vi "Calculate Mean Histogram Y Values.vi"(11 "Histograms":u32[][](array[numeric])) -> (3 "Mean Row Values":u8[](array[numeric]))   [LabVIEW 2015]
uses:
  <userlib>/_OpenG.lib/array/array.llb/Sort 1D Array (U32)__ogtk.vi
  <vilib>/Analysis/NI_AALBase.lvlib
panel:
  out "Waveform Graph":u32[][](graph)
  out "number of columns":i32
  out "number of rows":i32
  out "Sorted Pointers":i32[](array[numeric])
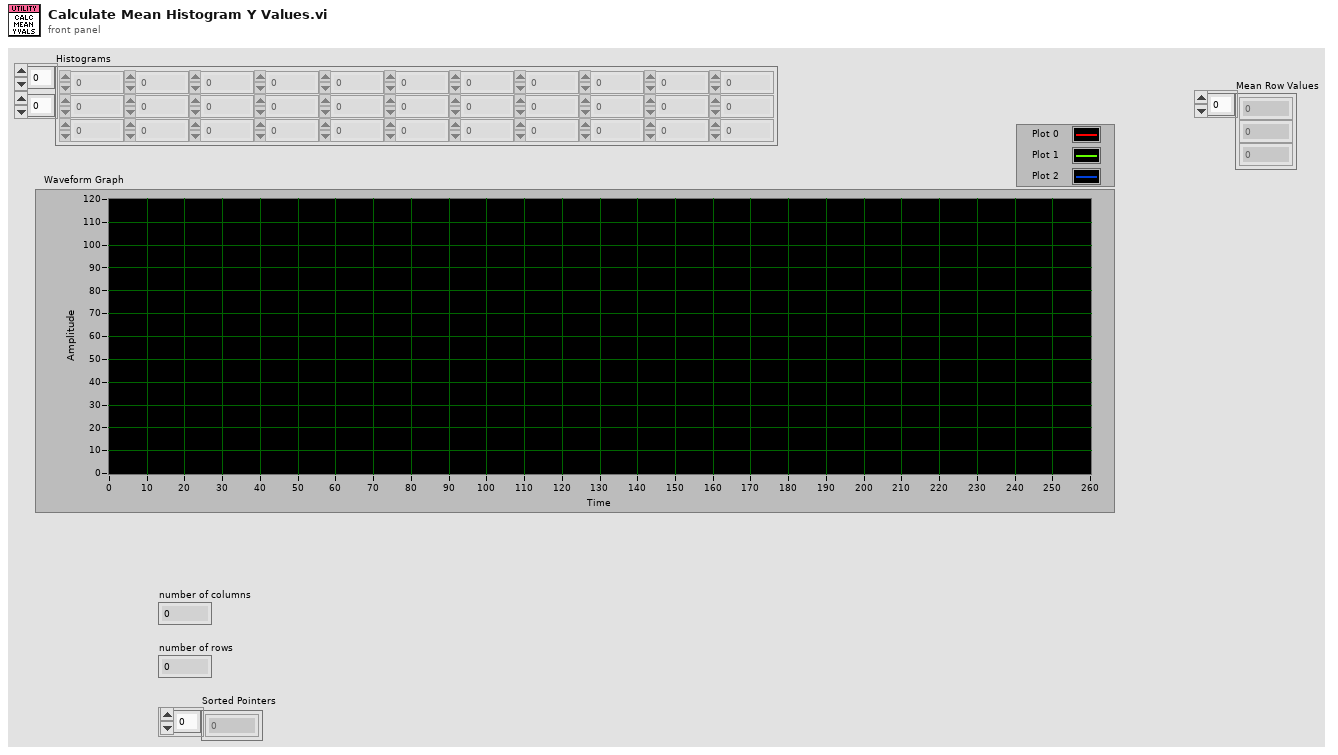
[diagram p1: front panel]
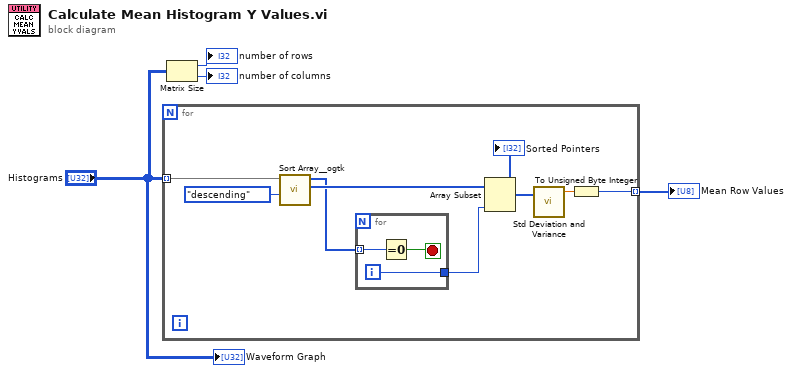
[diagram p0: block diagram]
diagram:
  n1 = for {
    tunnel: "Histograms" -> [w7] mode=indexing
    tunnel: [w8] -> w1 mode=indexing
    n2 = call-poly <userlib>:"Sort Array__ogtk.vi"("Order"=enum16{"ascending", "descending"}."descending", "Array in"=w7) -> ("Sorted Pointers"=w11:i32[], "Sorted Array out"=w6:u32[])  [unwired: 8 in]
    "Sorted Pointers" <- w11
    n3 = for {
      tunnel: w6 -> [w15] mode=indexing
      tunnel: [w13] -> w5
      i -> [w13]
      stop <- w14 stop-if-true
      n4 = Equal To 0?(x=w15) -> (x = 0?=w14:bool)
    }
    n5 = Array Subset(array=w11, length=w5) -> (w10:i32[])  [unwired: 1 in]
    n6 = call <vilib>:"Std Deviation and Variance.vi"("X"=w10) -> ("mean"=w9:dbl)  [unwired: 1 in, 2 out]
    n7 = To Unsigned Byte Integer(number=w9) -> (unsigned 8bit integer=w8:u8)
  }
  "Mean Row Values" <- w1
  n8 = Matrix Size(0:"Histograms") -> (1:→"number of rows":i32, 2:→"number of columns":i32)
  "Waveform Graph" <- "Histograms"
